vi "Matrix Vector Multiply.vi"(3 "n":i32, 4 "m":i32, 5 "B":sgl[](array[numeric]), 6 "A":sgl[](array[numeric])) -> (0 "C":sgl[](array[numeric]))   [LabVIEW 2020]
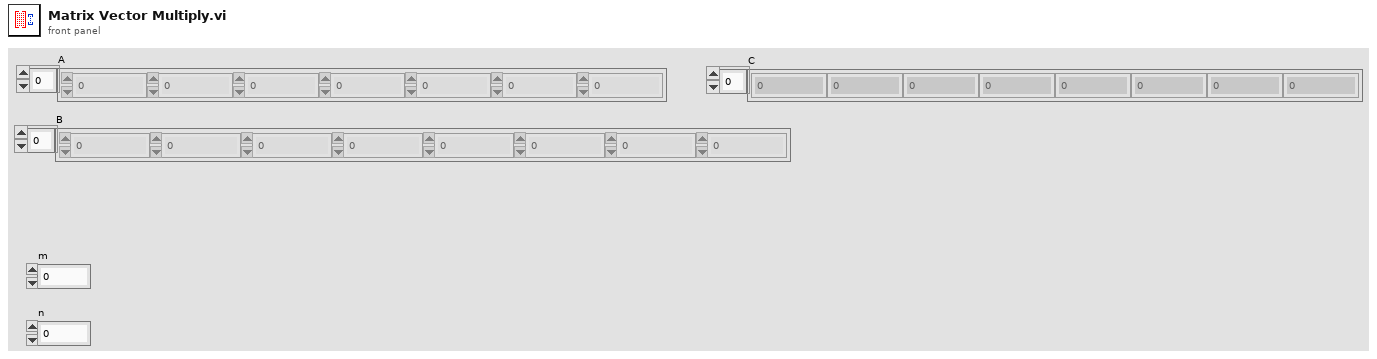
[diagram p1: front panel]
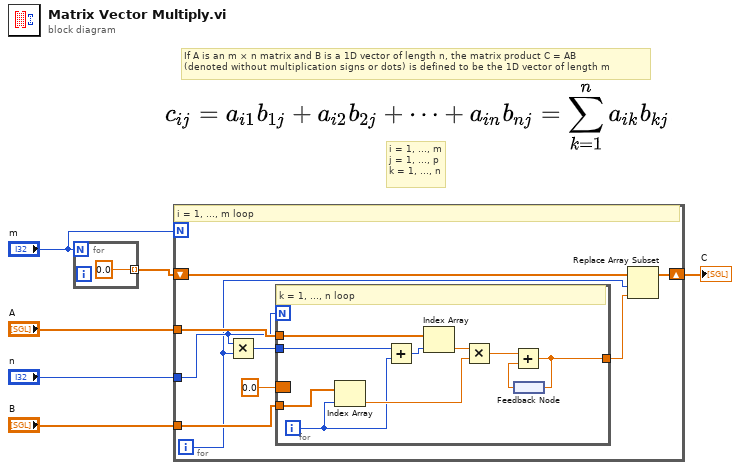
[diagram p0: block diagram]
diagram:
  # "If A is an m × n matrix and B is a 1D vector of length n, the matrix product C = AB \n(denoted without multiplication signs or dots) is defined to be the 1D vector of length m"
  # "i = 1, ..., m\nj = 1, ..., p\nk = 1, ..., n"
  n1 = for {
    N: "m" -> [_]
    tunnel: [sgl 0.0] -> w2 mode=indexing
  }
  n2 = for {
    N: "m" -> [_]
    tunnel: "B" -> [w16]
    tunnel: "A" -> [w13]
    tunnel: "n" -> [w12]
    shift-right: [w14] -> w4
    shift-left: w2 -> [w15]
    i -> [w8]
    # "i = 1, ..., m loop"
    n3 = Multiply(x=w12, y=w8) -> (x*y=w9:i32)
    n4 = for {
      N: w12 -> [_]
      tunnel: w13 -> [w26]
      tunnel: w9 -> [w18]
      tunnel: w16 -> [w25]
      tunnel: [w20] -> w10
      border: sgl 0.0 -> [_]
      i -> [w17]
      # "k = 1, ..., n loop"
      n5 = Index Array(array=w25, index=w17) -> (element=w23:sgl)
      n6 = Add(x=w18, y=w17) -> (x+y=w19:i32)
      n7 = Index Array(array=w26, index=w19) -> (element=w24:sgl)
      n8 = Multiply(x=w24, y=w23) -> (x*y=w22:sgl)
      n9 = feedback #1() -> (w21:sgl)
      n10 = Add(x=w22, y=w21) -> (x+y=w20:sgl)
      n11 = feedback-in #1(w20) -> ()
    }
    n12 = Replace Array Subset(array=w15, new element=w10, index=w8) -> (w14:sgl[])
  }
  "C" <- w4
